vi "Operator message space bar continue or usb gone.vi"(8 "error in (no error)":errorcluster, 10 "Message.Font:Size":u32=36, 11 "Message":string) -> (0 "error out":errorcluster)   [LabVIEW 2013]
uses:
  <vilib>/event_ctls.llb/eventvkey.ctl
  Test Globals/Global 1.vi
panel:
  # "Operator Message"
  # "Press SPACE BAR to continue"
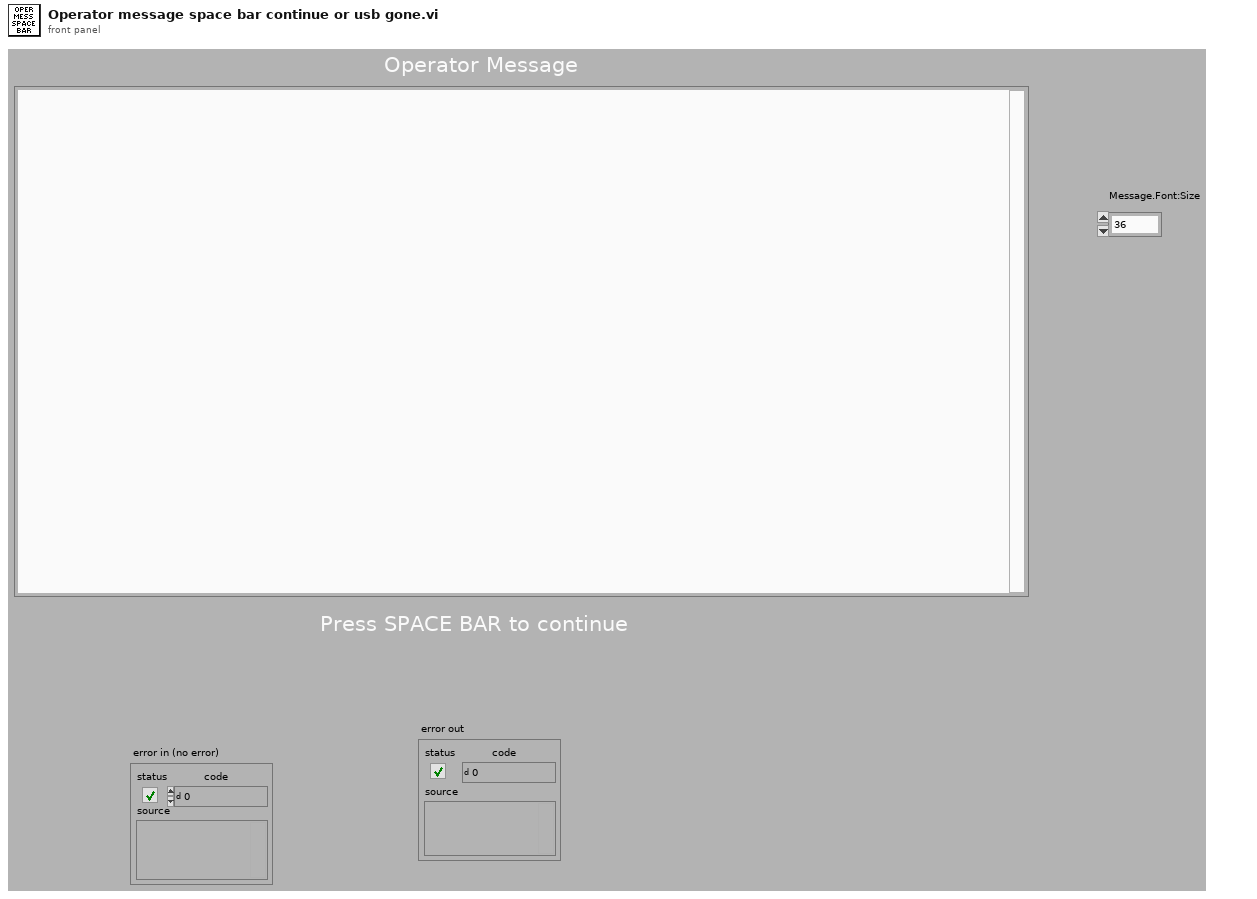
[diagram p1: front panel]
types:
  T1 = typedef "eventvkey.ctl" = enum16{"ASCII", "Enter", "Return", "Shift", "Ctrl", "Alt", "Cmd", "Opt", "Caps", "NumLock", "Clear", "Break", "Up", "Down", "Left", "Right", "Insert", "Delete", "Home", "End", "PageUp", "PageDown", "Escape", "Help", "Pause", "ScrollLock", "F1", "F2", "F3", "F4", "F5", "F6", "F7", "F8", "F9", "F10", "F11", "F12", "F13", "F14", "F15", "F16", "F17", "F18", "F19", "F20", "F21", "F22", "F23", "F24", "Play", "VolumeUp", "VolumeDown", "Mute", "Two Byte Char"}
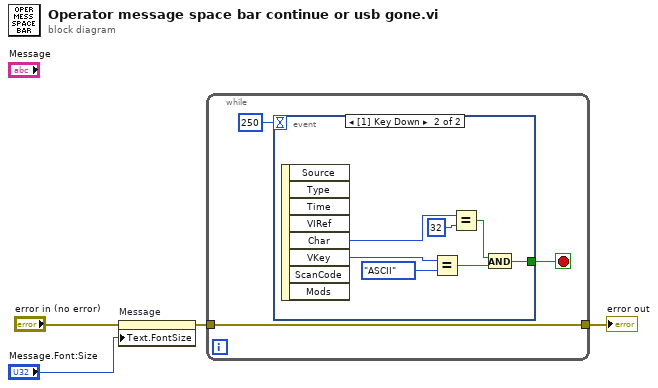
[diagram p0: block diagram]
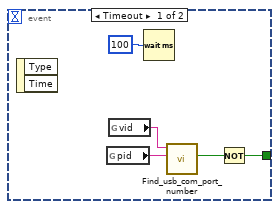
[diagram p2: hidden frame]
diagram:
  n1 = property on="Message" class="Str"(error in="error in (no error)", "Text.FontSize"="Message.Font:Size") -> (error out=w3:errorcluster)  [unwired: 1 in, 1 out]
  n2 = while {
    tunnel: [w6] -> w2
    tunnel: w3 -> [w6]
    stop <- w7 stop-if-true
    n3 = event shown="[1] Key Down" {
      selector: _ -> [_ _]
      dyn-events: _ -> [_ _]
      timeout: 250 -> [_ _]
      tunnel: [w8 w13] -> w7
      event Timeout {
        n4 = event-data() -> ()  [unwired: 1 in, 2 out]
        n5 = global read "Global 1.vi" "pid"() -> (w10:string)
        n6 = global read "Global 1.vi" "vid"() -> (w11:string)
        n7 = Wait (ms)(milliseconds to wait=u32 100) -> ()  [unwired: 1 out]
        n8 = call "Find_usb_com_port_number.vi"("Pid"=w10, "Vid"=w11) -> ("Found com port"=w9:bool)  [unwired: 5 in, 4 out]
        n9 = Not(x=w9) -> (.not. x?=w8:bool)
      }
      event Key Down {
        n10 = event-data() -> ("Char"=w19:i16, "VKey"=w17:T1)  [unwired: 1 in, 6 out]
        n11 = Equal?(x=w17, y=eventvkey."ASCII" ("VKey")) -> (x = y?=w14:bool)
        n12 = Equal?(x=w19, y=i16 32) -> (x = y?=w15:bool)
        n13 = And(x=w15, y=w14) -> (x .and. y?=w13:bool)
      }
    }
  }
  "error out" <- w2
